vi "Acquisition.vi"(0 ".NET (Reference)":refnum<k24>, 5 "Camera Param. Control Cluster":T1, 7 "Bits/Pixel in":i32, 9 "Pupil Param. Calc. Data Cluster":T2={"img_rows"=0, "img_cols"=0, "AT"=43, "GB"=17, "N_pts"=100}, 11 "Error In":errorcluster) -> (4 ".NET (Reference)":refnum<k24>, 6 "Image To Save":u8[][](array[numeric]), 8 "Framerate":dbl, 14 "Camera Image":picture, 15 "Error Out":errorcluster)   [LabVIEW 2021]
uses:
  C:/Program Files/Thorlabs/Scientific Imaging/ThorCam/uc480DotNet.dll
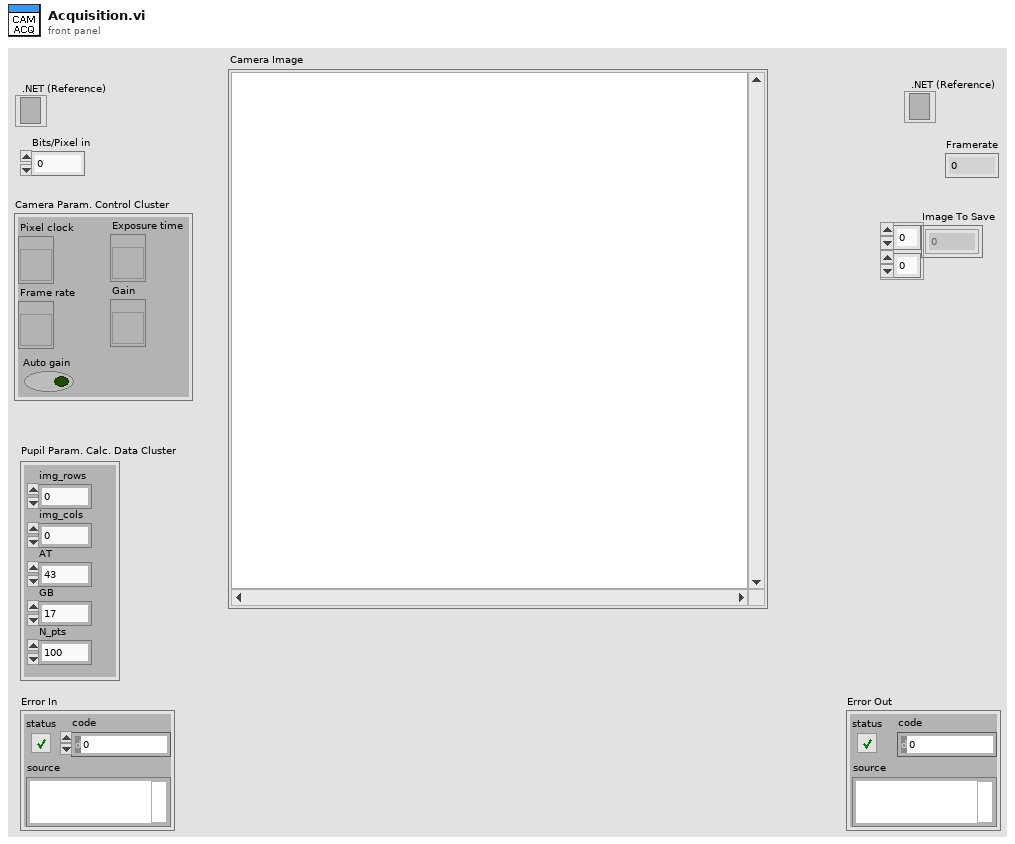
[diagram p1: front panel]
types:
  T1 = cluster{"Pixel clock":refnum<vi>, "Frame rate":refnum<vi>, "Exposure time":refnum<vi>, "Gain":refnum<vi>, "Auto gain":bool}
  T2 = cluster{"img_rows":u16, "img_cols":u16, "AT":u8, "GB":u8, "N_pts":u8}
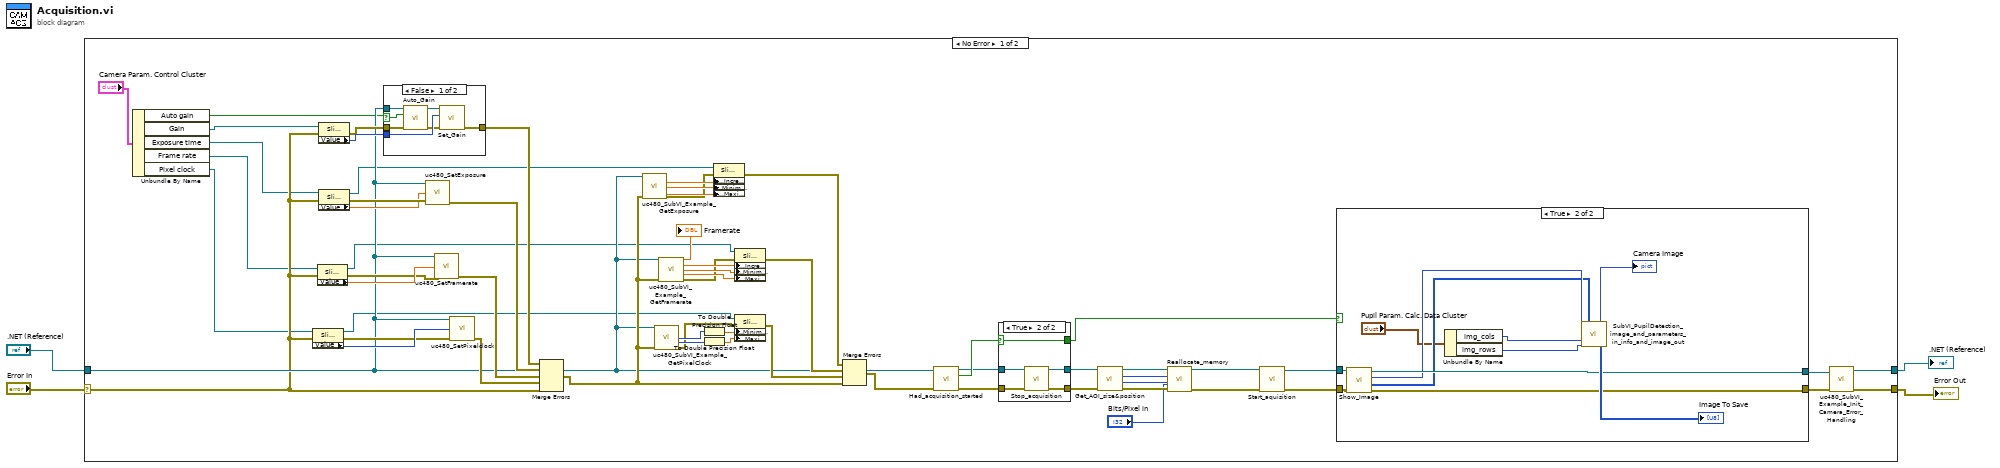
[diagram p0: block diagram]
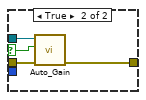
[diagram p4: hidden frame]
diagram:
  n1 = case shown="No Error" "Error In" {
    selector: "Error In" -> [w13 w99]
    tunnel: [w59 w99] -> w4
    tunnel: ".NET (Reference)" -> [w14 w98]
    tunnel: [w47 w98] -> w1
    frame No Error {
      n2 = Unbundle By Name("Camera Param. Control Cluster") -> ("Auto gain"=w12:bool, "Gain"=w11:refnum<vi>, "Exposure time"=w10:refnum<vi>, "Frame rate"=w9:refnum<vi>, "Pixel clock"=w8:refnum<vi>)
      n3 = property class="Slide (strict)"(reference=w8, error in=w13) -> (reference out=w7:refnum<vi>, error out=w49:errorcluster, "Value"=w57:i32)
      n4 = property class="Slide (strict)"(reference=w9, error in=w13) -> (reference out=w6:refnum<vi>, error out=w55:errorcluster, "Value"=w56:dbl)
      n5 = property class="Slide (strict)"(reference=w11, error in=w13) -> (error out=w54:errorcluster, "Value"=w58:i32)  [unwired: 1 out]
      n6 = property class="Slide (strict)"(reference=w10, error in=w13) -> (reference out=w5:refnum<vi>, error out=w53:errorcluster, "Value"=w52:dbl)
      n7 = case shown="False" w12 {
        selector: w12 -> [w93 w97]
        tunnel: [w90 w96] -> w15
        tunnel: w58 -> [w92 _]
        tunnel: w54 -> [w89 w95]
        tunnel: w14 -> [w88 w94]
        frame False {
          n8 = call "Auto_Gain.vi"("error in (no error)"=w89, "Auto gain"=w93, "uc480.Camera"=w88) -> ("error out"=w91:errorcluster, "uc480.Camera"=w87:refnum<k24>)  [unwired: 7 in]
          n9 = call "Set_Gain.vi"("error in (no error)"=w91, "Gain"=w92, "uc480.Camera"=w87) -> ("error out"=w90:errorcluster)  [unwired: 8 in]
        }
        frame True {
          n10 = call "Auto_Gain.vi"("error in (no error)"=w95, "Auto gain"=w97, "uc480.Camera"=w94) -> ("error out"=w96:errorcluster)  [unwired: 7 in, 1 out]
        }
      }
      n11 = call "uc480_SetExposure.vi"("uc480.Camera"=w14, "Exposure time"=w52, "Error In"=w53) -> ("Error out"=w16:errorcluster)  [unwired: 12 in]
      n12 = call "uc480_SetFramerate.vi"("uc480.Camera"=w14, "Frame rate"=w56, "Error In"=w55) -> ("Error out"=w17:errorcluster)  [unwired: 12 in]
      n13 = call "uc480_SetPixelclock.vi"("uc480.Camera"=w14, "Pixel clock"=w57, "Error In"=w49) -> ("Error out"=w18:errorcluster)  [unwired: 12 in]
      n14 = Merge Errors(w15, w16, w17, w18, w13) -> (w19:errorcluster)
      n15 = call "uc480_SubVI_Example_GetExposure.vi"("uc480.Camera"=w14, "Error In"=w19) -> ("Inc"=w25:dbl, "Min"=w24:dbl, "Max"=w23:dbl, "Error out"=w22:errorcluster)  [unwired: 9 in, 1 out]
      n16 = call "uc480_SubVI_Example_GetPixelClock.vi"("uc480.Camera"=w14, "Error In"=w19) -> ("Min"=w33:i32, "Max"=w32:i32, "error out"=w31:errorcluster)  [unwired: 9 in, 2 out]
      n17 = call "uc480_SubVI_Example_GetFramerate.vi"("uc480.Camera"=w14, "Error In"=w19) -> ("Framerate"=→"Framerate":dbl, "Inc"=w29:dbl, "Min"=w28:dbl, "Max"=w27:dbl, "error out"=w26:errorcluster)  [unwired: 9 in]
      n18 = To Double Precision Float(number=w33) -> (double precision float=w50:dbl)
      n19 = To Double Precision Float(number=w32) -> (double precision float=w51:dbl)
      n20 = property on="Property Node" class="Slide (strict)"(reference=w5, error in=w22, "Scale.Increment"=w25, "Scale.Minimum"=w24, "Scale.Maximum"=w23) -> (error out=w20:errorcluster)  [unwired: 1 out]
      n21 = property class="Slide (strict)"(reference=w6, error in=w26, "Scale.Increment"=w29, "Scale.Minimum"=w28, "Scale.Maximum"=w27) -> (error out=w21:errorcluster)  [unwired: 1 out]
      n22 = property class="Slide (strict)"(reference=w7, error in=w31, "Scale.Minimum"=w50, "Scale.Maximum"=w51) -> (error out=w30:errorcluster)  [unwired: 1 out]
      n23 = Merge Errors(w20, w21, w30, w19) -> (w34:errorcluster)
      n24 = call "Had_acquisition_started.vi"("error in (no error)"=w34, "uc480.Camera"=w14) -> ("error out"=w62:errorcluster, "bValue"=w38:bool, "uc480.Camera"=w35:refnum<k24>)  [unwired: 6 in]
      n25 = case shown="True" w38 {
        selector: w38 -> [w80 w84]
        tunnel: w62 -> [w81 w86]
        tunnel: [w81 w85] -> w39
        tunnel: [w80 w84] -> w37
        tunnel: [w79 w83] -> w36
        tunnel: w35 -> [w79 w82]
        frame False {
        }
        frame True {
          n26 = call "Stop_acquisition.vi"("error in (no error)"=w86, "uc480.Camera"=w82) -> ("error out"=w85:errorcluster, "uc480.Camera"=w83:refnum<k24>)  [unwired: 8 in]
        }
      }
      n27 = call "Get_AOI_size&position.vi"("error in (no error)"=w39, "uc480.Camera"=w36) -> ("error out"=w63:errorcluster, "s32Height"=w40:i32, "s32Width"=w41:i32, "uc480.Camera"=w42:refnum<k24>)  [unwired: 5 in]
      n28 = call "Reallocate_memory.vi"("uc480.Camera"=w42, "s32Width"=w41, "s32Height"=w40, "Bits/Pixel in"="Bits/Pixel in", "error in (no error)"=w63) -> ("uc480.Camera"=w44:refnum<k24>, "error out"=w64:errorcluster)  [unwired: 9 in]
      n29 = call "Start_aquisition.vi"("error in (no error)"=w64, "uc480.Camera"=w44) -> ("error out"=w65:errorcluster, "uc480.Camera"=w45:refnum<k24>)  [unwired: 8 in]
      n30 = case shown="True" w37 {
        tunnel: w65 -> [w67 w78]
        tunnel: [w67 w68] -> w60
        tunnel: [w66 w73] -> w46
        tunnel: w45 -> [w66 w72]
        frame False {
        }
        frame True {
          n31 = call "Show_Image.vi"("error in (no error)"=w78, "uc480.Camera"=w72) -> ("error out"=w68:errorcluster, "u8Image"=w70:u8[], "Image"=w71:picture, "uc480.Camera"=w73:refnum<k24>)  [unwired: 6 in]
          n32 = Unbundle By Name("Pupil Param. Calc. Data Cluster") -> ("img_cols"=w75:u16, "img_rows"=w74:u16)
          n33 = call "SubVI_PupilDetection_image_and_parameters_in_info_and_image_out.vi"("Image"=w71, "img_cols"=w75, "img_rows"=w74, "u8Image"=w70) -> ("output image"=→"Camera Image":picture, "Image to save"=→"Image To Save":u8[][])  [unwired: 14 in]
        }
      }
      n34 = call "uc480_SubVI_Example_Init_Camera_Error_Handling.vi"("Error In"=w60, "uc480.Camera"=w46) -> ("Error Out"=w59:errorcluster, "uc480.Camera"=w47:refnum<k24>)  [unwired: 8 in]
    }
    frame Error {
    }
  }
  "Error Out" <- w4
  ".NET (Reference)" <- w1
